vi "Add Gauge Hi Lo Alarms.vi"(6 "Enable":bool, 7 "Action":T1(ring)=enum."Update Flow Limit", 8 "Current Flow Limits":cluster{"Low Limit":dbl, "Hi Limit":dbl}, 9 "Limits":cluster{"Low Limit":dbl, "Hi Limit":dbl}[](array[cluster]), 10 "reference":refnum<vi>) -> ()   [LabVIEW 2018]
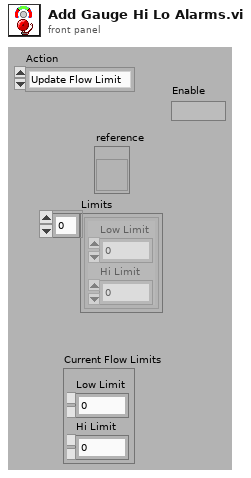
[diagram p1: front panel]
types:
  T1 = enum16{"Init", "Add Alarm Limits", "Update Flow Limit", "Check for Alarm", "Clear Alarms"}
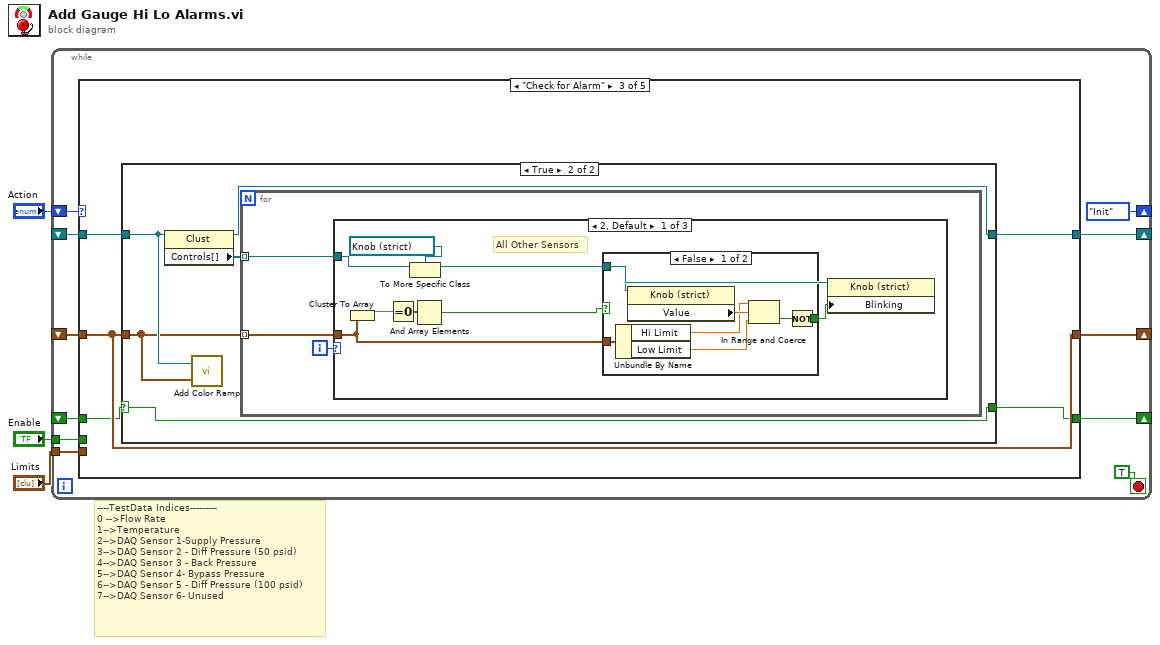
[diagram p0: block diagram]
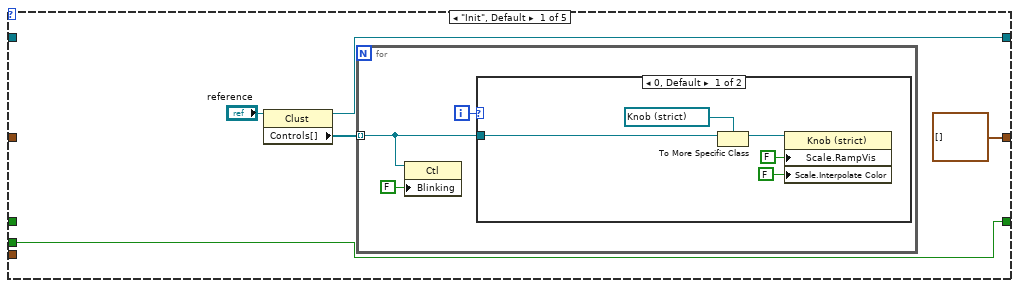
[diagram p2: hidden frame]
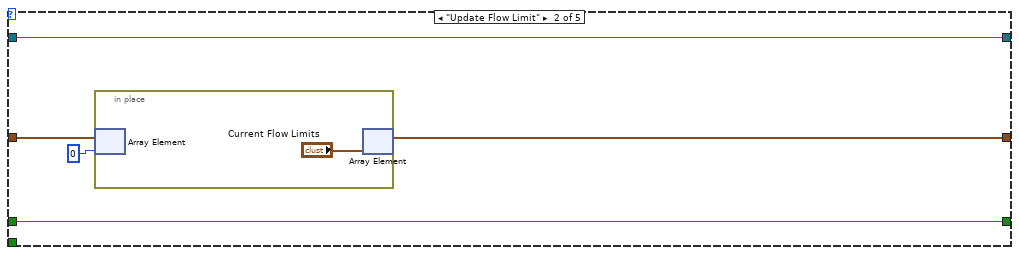
[diagram p4: hidden frame]
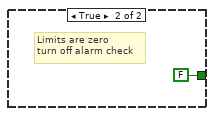
[diagram p6: hidden frame]
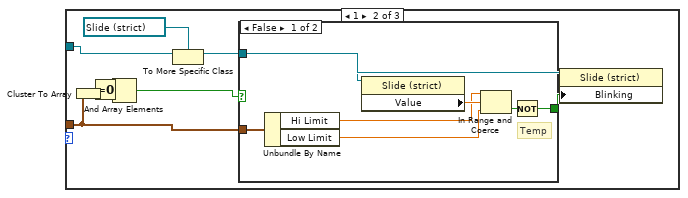
[diagram p7: hidden frame]
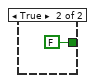
[diagram p8: hidden frame]
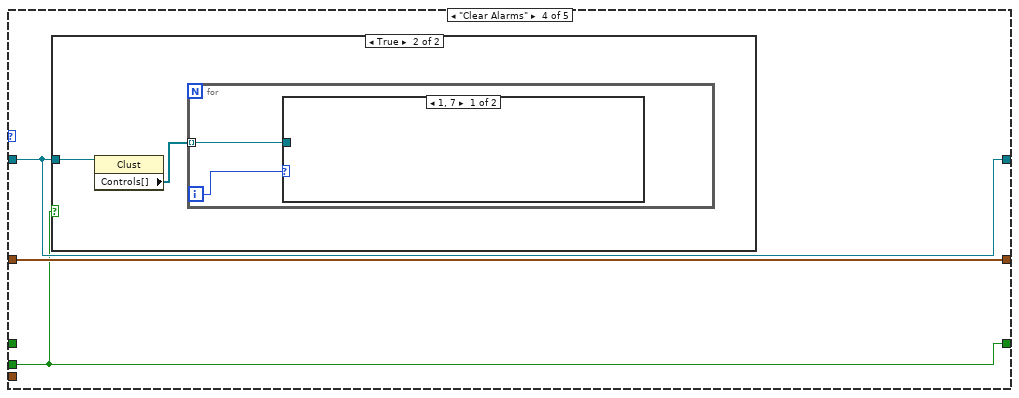
[diagram p10: hidden frame]
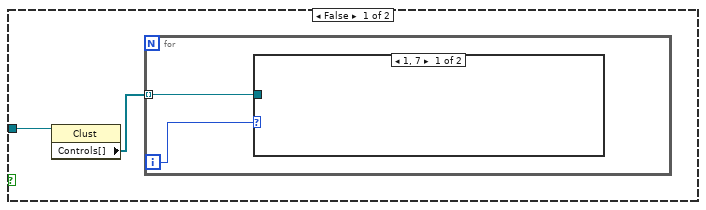
[diagram p11: hidden frame]
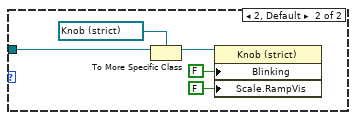
[diagram p12: hidden frame]
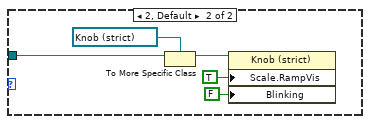
[diagram p13: hidden frame]
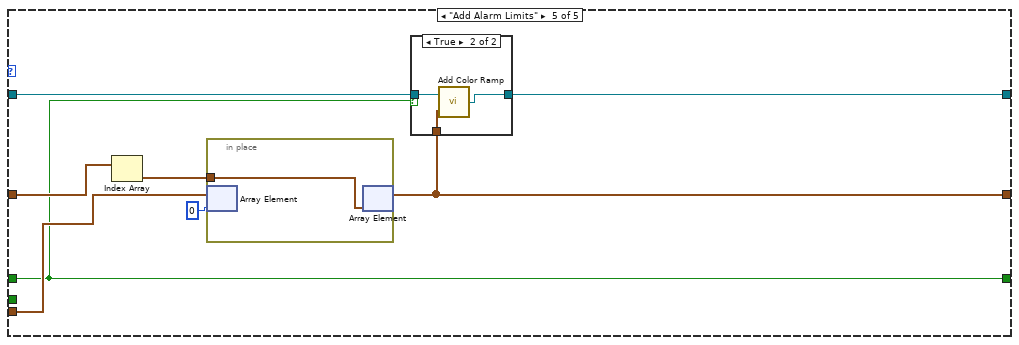
[diagram p14: hidden frame]
diagram:
  # "----TestData Indices---------\n0 -->Flow Rate\n1-->Temperature\n2-->DAQ Sensor 1-Supply Pressure\n3-->DAQ Sensor 2 - Diff Pressure (50 psid)\n4-->DAQ Sensor 3 - Back Pressure\n5-->DAQ Sensor 4- Bypass Pressure\n6-->DAQ Sensor 5 - Diff Pressure (100 psid)\n7-->DAQ Sensor 6- Unused"
  n1 = while {
    shift-right: [T1."Init"] -> _
    shift-left: "Action" -> [w14]
    shift-right: [w13] -> _
    shift-left: _ -> [w12]
    shift-right: [w11] -> _
    shift-left: _ -> [w9]
    shift-right: [w7] -> _
    shift-left: _ -> [w6]
    tunnel: "Enable" -> [w5]
    tunnel: "Limits" -> [w4]
    stop <- TRUE stop-if-true
    n2 = case shown="\"Check for Alarm\"" w14 {
      tunnel: [w16 w32 w36 w82 w108] -> w13
      tunnel: w12 -> [_ w32 w38 w82 w109]
      tunnel: [cluster{"Low Limit":dbl, "Hi Limit":dbl}[] [] ("Limits") w30 w37 w83 w107] -> w11
      tunnel: w9 -> [_ w31 w37 w83 w106]
      tunnel: [w15 w28 w34 w81 w102] -> w7
      tunnel: w6 -> [_ w28 w35 _ w102]
      tunnel: w5 -> [w15 _ _ w81 _]
      tunnel: w4 -> [_ _ _ _ w105]
      frame "Init", Default {
        n3 = property on="Property Node" class="Clust"(reference="reference") -> (reference out=w16:refnum<vi>, "Controls[]"=w17:refnum<vi>[])  [unwired: 1 in, 1 out]
        n4 = for {
          tunnel: w17 -> [w21] mode=indexing
          i -> [w22]
          n5 = property class="Ctl"(reference=w21, "Blinking"=FALSE) -> ()  [unwired: 1 in, 2 out]
          n6 = case shown="0, Default" w22 {
            tunnel: w21 -> [w27 _]
            frame 0, Default {
              n7 = To More Specific Class(target class=refnum<vi> refnum ("Knob Refnum"), reference=w27) -> (specific class reference=w26:refnum<vi>)  [unwired: 1 in, 1 out]
              n8 = property on="Property Node" class="Knob (strict)"(reference=w26, "Scale.RampVis"=FALSE ("Scale.Ramp Visible"), "Scale.Interpolate Color"=FALSE) -> ()  [unwired: 1 in, 2 out]
            }
            frame 7 {
            }
          }
        }
      }
      frame "Update Flow Limit" {
        n9 = in-place {
          n10 = in-place-array #1(w31, 0) -> ()  [unwired: 1 out]
          n11 = in-place-array #1("Current Flow Limits") -> (w30:cluster{"Low Limit":dbl, "Hi Limit":dbl}[])  [unwired: 1 out]
        }
      }
      frame "Check for Alarm" {
        n12 = case shown="True" w35 {
          selector: w35 -> [w39 w43]
          tunnel: w38 -> [w40 w42]
          tunnel: w37 -> [_ w41]
          tunnel: [w40 w44] -> w36
          tunnel: [w39 w43] -> w34
          frame False {
          }
          frame True {
            n13 = property on="Property Node" class="Clust"(reference=w42) -> (reference out=w44:refnum<vi>, "Controls[]"=w45:refnum<vi>[])  [unwired: 1 in, 1 out]
            n14 = call "Add Color Ramp.vi"("Limits"=w41, "reference in"=w42) -> ()  [unwired: 1 out]
            n15 = for {
              tunnel: w45 -> [w47] mode=indexing
              tunnel: w41 -> [w46] mode=indexing
              i -> [w48]
              n16 = case shown="2, Default" w48 {
                tunnel: w47 -> [w56 w70 _]
                tunnel: w46 -> [w55 w66 _]
                frame 2, Default {
                  # "All Other Sensors"
                  n17 = Cluster To Array(cluster=w55) -> (array=w54:dbl[])
                  n18 = Equal To 0?(x=w54) -> (x = 0?=w53:bool[])
                  n19 = To More Specific Class(target class=refnum<vi> refnum ("Knob Refnum"), reference=w56) -> (specific class reference=w50:refnum<vi>)  [unwired: 1 in, 1 out]
                  n20 = And Array Elements(Boolean array=w53) -> (logical AND=w49:bool)
                  n21 = case shown="False" w49 {
                    tunnel: w55 -> [w63 _]
                    tunnel: [w62 FALSE] -> w52
                    tunnel: w50 -> [w57 _]
                    frame False {
                      n22 = Unbundle By Name(w63) -> ("Hi Limit"=w59:dbl, "Low Limit"=w58:dbl)
                      n23 = property on="Property Node" class="Knob (strict)"(reference=w57) -> ("Value"=w60:dbl)  [unwired: 1 in, 2 out]
                      n24 = In Range and Coerce(upper limit=w59, x=w60, lower limit=w58) -> (In Range?=w61:bool)  [unwired: 1 out]
                      n25 = Not(x=w61) -> (.not. x?=w62:bool)
                    }
                    frame True {
                      # "Limits are zero \nturn off alarm check"
                    }
                  }
                  n26 = property on="Property Node" class="Knob (strict)"(reference=w50, "Blinking"=w52) -> ()  [unwired: 1 in, 2 out]
                }
                frame 1 {
                  n27 = Cluster To Array(cluster=w66) -> (array=w68:dbl[])
                  n28 = Equal To 0?(x=w68) -> (x = 0?=w67:bool[])
                  n29 = And Array Elements(Boolean array=w67) -> (logical AND=w65:bool)
                  n30 = To More Specific Class(target class=refnum<vi> refnum ("Fuel Temp"), reference=w70) -> (specific class reference=w71:refnum<vi>)  [unwired: 1 in, 1 out]
                  n31 = case shown="False" w65 {
                    tunnel: [w79 FALSE] -> w72
                    tunnel: w71 -> [w76 _]
                    tunnel: w66 -> [w73 _]
                    frame False {
                      # "Temp"
                      n32 = Unbundle By Name(w73) -> ("Hi Limit"=w74:dbl, "Low Limit"=w75:dbl)
                      n33 = property on="Property Node" class="Slide (strict)"(reference=w76) -> ("Value"=w77:dbl)  [unwired: 1 in, 2 out]
                      n34 = In Range and Coerce(upper limit=w74, x=w77, lower limit=w75) -> (In Range?=w78:bool)  [unwired: 1 out]
                      n35 = Not(x=w78) -> (.not. x?=w79:bool)
                    }
                    frame True {
                    }
                  }
                  n36 = property on="Property Node" class="Slide (strict)"(reference=w71, "Blinking"=w72) -> ()  [unwired: 1 in, 2 out]
                }
                frame 7 {
                }
              }
            }
          }
        }
      }
      frame "Clear Alarms" {
        n37 = case shown="True" w81 {
          tunnel: w82 -> [w85 w94]
          frame False {
            n38 = property on="Property Node" class="Clust"(reference=w85) -> ("Controls[]"=w84:refnum<vi>[])  [unwired: 1 in, 2 out]
            n39 = for {
              tunnel: w84 -> [w87] mode=indexing
              i -> [w86]
              n40 = case shown="1, 7" w86 {
                tunnel: w87 -> [_ w91]
                frame 1, 7 {
                }
                frame 2, Default {
                  n41 = To More Specific Class(target class=refnum<vi> refnum ("Knob Refnum"), reference=w91) -> (specific class reference=w89:refnum<vi>)  [unwired: 1 in, 1 out]
                  n42 = property on="Property Node" class="Knob (strict)"(reference=w89, "Blinking"=FALSE, "Scale.RampVis"=FALSE ("Scale.Ramp Visible")) -> ()  [unwired: 1 in, 2 out]
                }
              }
            }
          }
          frame True {
            n43 = property on="Property Node" class="Clust"(reference=w94) -> ("Controls[]"=w93:refnum<vi>[])  [unwired: 1 in, 2 out]
            n44 = for {
              tunnel: w93 -> [w96] mode=indexing
              i -> [w95]
              n45 = case shown="1, 7" w95 {
                tunnel: w96 -> [_ w101]
                frame 1, 7 {
                }
                frame 2, Default {
                  n46 = To More Specific Class(target class=refnum<vi> refnum ("Knob Refnum"), reference=w101) -> (specific class reference=w99:refnum<vi>)  [unwired: 1 in, 1 out]
                  n47 = property on="Property Node" class="Knob (strict)"(reference=w99, "Scale.RampVis"=TRUE ("Scale.Ramp Visible"), "Blinking"=FALSE) -> ()  [unwired: 1 in, 2 out]
                }
              }
            }
          }
        }
      }
      frame "Add Alarm Limits" {
        n48 = Index Array(array=w106) -> (element=w103:cluster{"Low Limit":dbl, "Hi Limit":dbl})  [unwired: 1 in]
        n49 = in-place {
          in-place-border: w103 -> [w114]
          n50 = in-place-array #2(w105, 0) -> ()  [unwired: 1 out]
          n51 = in-place-array #2(w114) -> (w107:cluster{"Low Limit":dbl, "Hi Limit":dbl}[])  [unwired: 1 out]
        }
        n52 = case shown="True" w102 {
          tunnel: w109 -> [w110 w113]
          tunnel: [w110 w112] -> w108
          tunnel: w107 -> [_ w111]
          frame False {
          }
          frame True {
            n53 = call "Add Color Ramp.vi"("Limits"=w111, "reference in"=w113) -> ("reference out"=w112:refnum<vi>)
          }
        }
      }
    }
  }
